vi "GetKey.vi"(10 "x":u16 format="%.0x") -> (2 "KEY":u8[](array[numeric]) format="%.0x")   [LabVIEW 2018]
panel:
  out "lo(x)":u8 format="%.0x"
  out "hi(x)":u8 format="%.0x"
  out "十六进制整型字符串":string
  out "y":u16 format="%.0x"
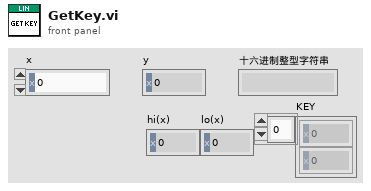
[diagram p1: front panel]
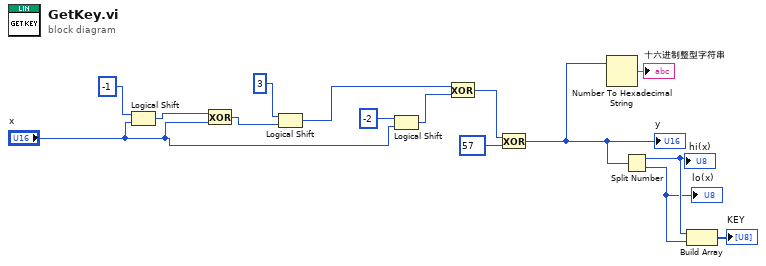
[diagram p0: block diagram]
diagram:
  n1 = Logical Shift(y=i16 -1, x="x") -> (x << y=w14:u16)
  n2 = Exclusive Or(1:"x", 2:w14) -> (0:w13:u16)
  n3 = Logical Shift(y=i16 3, x=w13) -> (x << y=w8:u16)
  n4 = Logical Shift(y=i16 -2, x="x") -> (x << y=w9:u16)
  n5 = Exclusive Or(1:w9, 2:w8) -> (0:w7:u16)
  n6 = Exclusive Or(1:u16 57 ("y"), 2:w7) -> (0:w4:u16)
  "y" <- w4
  n7 = Number To Hexadecimal String(2:w4) -> (0:→"十六进制整型字符串":string)  [unwired: 1 in]
  n8 = Split Number(x=w4) -> (hi(x)=w3:u8, lo(x)=w2:u8)
  "hi(x)" <- w3
  "lo(x)" <- w2
  n9 = Build Array(w3, w2) -> (→"KEY":u8[])
